vi "Wait for AT cmds ready.vi"() -> ()   [LabVIEW 2013]
panel:
  out "error out":errorcluster
  in  "error in (no error)":errorcluster
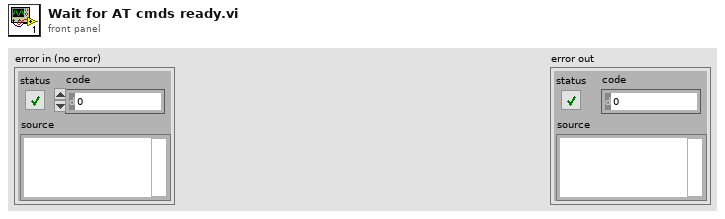
[diagram p1: front panel]
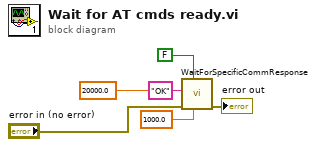
[diagram p0: block diagram]
diagram:
  n1 = call "WaitForSpecificCommResponse.vi"("Check period (msecs)"=1000.0, "Display err mess?"=FALSE, "error in (no error)"="error in (no error)", "Timeout (mSecs)"=20000.0, "Wait for"="OK") -> ("error out"=→"error out":errorcluster)  [unwired: 2 in, 4 out]
